vi "FreqToFTW.vi"(1 "Frequency":dbl) -> (0 "FTW [32bit]":u32)   [LabVIEW 2013]
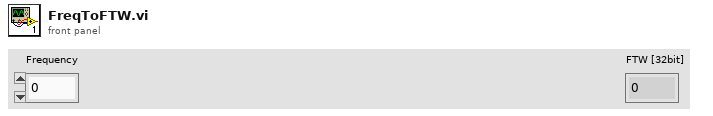
[diagram p1: front panel]
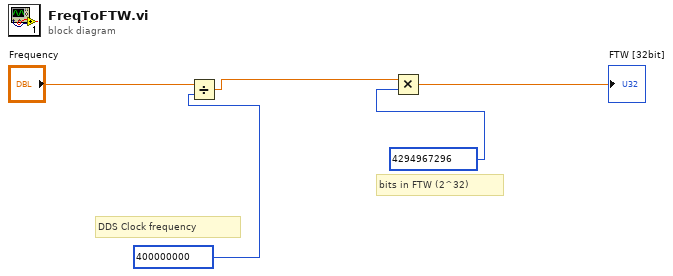
[diagram p0: block diagram]
diagram:
  # "bits in FTW (2^32)"
  # "DDS Clock frequency"
  n1 = Divide(x="Frequency", y=400000000) -> (x/y=w3:dbl)
  n2 = Multiply(x=w3, y=u64 4294967296) -> (x*y=→"FTW [32bit]":dbl)
